vi "main(Test DQMH modules).vi"() -> ()   [LabVIEW 2018, in "Application.lvlib"] (continued)
      tunnel: [w268 w1259 w1272 w1282 w1301 w1434 w1477 w1534 w1590 w1602 w1614 w1623 w1648 w1678 w1708 w1775 w1790 w1813 w1836 w1860 w1894 w1913 w1932 w1951 w1983 w2014 w2039 w2068 w2104 w2124 w2147 w2181 w2198 w2224 w2256 w2294 w2331 w2381 w2418 w2465 w2520 w2593 w2663 w2734 w2805 w2876 w2947 w3018 w3090 w3163 w3239 w3318 w3398 w3479 w3561 w3607 w3648 w3689 w3730 w3771 w3812 w3853 w3894 w3935 w3976 w4017 w4058 w4099 w4140 w4181 w4222 w4263 w4304 w4345 w4386 w4427 w4468 w4509 w4550 w4591 w4632 w4673 w4714 w4755 w4796 w4837 w4878 w4919 w4960 w5001 w5042 w5083 w5124 w5165 w5206 w5247 w5288 w5329 w5370 w5411 w5452 w5493 w5534 w5575 w5616 w5657 w5698 w5739 w5780 w5821 w5862 w5903 w5944 w5985 w6026 w6064 1 ("DUT channel (1-11)") 1 ("DUT channel (1-11)") 1 ("DUT channel (1-11)") 1 ("DUT channel (1-11)") 1 ("DUT channel (1-11)") 1 ("DUT channel (1-11)") 2 ("DUT channel (1-11)") 2 ("DUT channel (1-11)") 2 ("DUT channel (1-11)") 2 ("DUT channel (1-11)") 2 ("DUT channel (1-11)") 2 ("DUT channel (1-11)") 3 ("DUT channel (1-11)") 3 ("DUT channel (1-11)") 3 ("DUT channel (1-11)") 3 ("DUT channel (1-11)") 3 ("DUT channel (1-11)") 3 ("DUT channel (1-11)") 4 ("DUT channel (1-11)") 4 ("DUT channel (1-11)") 4 ("DUT channel (1-11)") 4 ("DUT channel (1-11)") 4 ("DUT channel (1-11)") 4 ("DUT channel (1-11)") 5 ("DUT channel (1-11)") 5 ("DUT channel (1-11)") 5 ("DUT channel (1-11)") 5 ("DUT channel (1-11)") 5 ("DUT channel (1-11)") 5 ("DUT channel (1-11)") 6 ("DUT channel (1-11)") 6 ("DUT channel (1-11)") 6 ("DUT channel (1-11)") 6 ("DUT channel (1-11)") 6 ("DUT channel (1-11)") 6 ("DUT channel (1-11)") 7 ("DUT channel (1-11)") 7 ("DUT channel (1-11)") 7 ("DUT channel (1-11)") 7 ("DUT channel (1-11)") 7 ("DUT channel (1-11)") 7 ("DUT channel (1-11)") 8 ("DUT channel (1-11)") 8 ("DUT channel (1-11)") 8 ("DUT channel (1-11)") 8 ("DUT channel (1-11)") 8 ("DUT channel (1-11)") 8 ("DUT channel (1-11)") 9 ("DUT channel (1-11)") 9 ("DUT channel (1-11)") 9 ("DUT channel (1-11)") 9 ("DUT channel (1-11)") 9 ("DUT channel (1-11)") 9 ("DUT channel (1-11)") 10 ("DUT channel (1-11)") 10 ("DUT channel (1-11)") 10 ("DUT channel (1-11)") 10 ("DUT channel (1-11)") 10 ("DUT channel (1-11)") 10 ("DUT channel (1-11)")] -> w237
      tunnel: w236 -> [w269 w1259 w1272 w1282 w1301 w1434 w1477 w1534 w1590 w1602 w1614 w1623 w1648 w1678 w1708 w1775 w1790 w1813 w1836 w1860 w1894 w1913 w1932 w1951 w1983 w2014 w2039 w2068 w2104 w2124 w2147 w2181 w2198 w2224 w2256 w2294 w2331 w2381 w2418 w2465 _ _ _ _ _ _ _ _ _ _ _ _ _ _ _ w3607 w3648 w3689 w3730 w3771 w3812 w3853 w3894 w3935 w3976 w4017 w4058 w4099 w4140 w4181 w4222 w4263 w4304 w4345 w4386 w4427 w4468 w4509 w4550 w4591 w4632 w4673 w4714 w4755 w4796 w4837 w4878 w4919 w4960 w5001 w5042 w5083 w5124 w5165 w5206 w5247 w5288 w5329 w5370 w5411 w5452 w5493 w5534 w5575 w5616 w5657 w5698 w5739 w5780 w5821 w5862 w5903 w5944 w5985 w6026 w6064 _ _ _ _ _ _ _ _ _ _ _ _ _ _ _ _ _ _ _ _ _ _ _ _ _ _ _ _ _ _ _ _ _ _ _ _ _ _ _ _ _ _ _ _ _ _ _ _ _ _ _ _ _ _ _ _ _ _ _ _]
      tunnel: [w266 w1258 w1271 w1281 w1303 w1422 w1476 w1533 w1589 w1601 w1613 w1622 w1647 w1677 w1707 w1774 w1789 w1812 w1835 w1859 w1893 w1912 w1931 w1950 w1982 w2013 w2038 w2067 w2103 w2123 w2146 w2180 w2197 w2223 w2259 w2293 w2330 w2380 w2409 w2464 w2498 w2592 w2662 w2733 w2804 w2875 w2946 w3017 w3089 w3162 w3238 w3317 w3397 w3478 w3560 w3602 w3644 w3685 w3726 w3767 w3811 w3849 w3890 w3931 w3972 w4013 w4054 w4095 w4136 w4177 w4218 w4258 w4302 w4341 w4382 w4423 w4464 w4505 w4546 w4587 w4628 w4669 w4710 w4751 w4791 w4833 w4874 w4915 w4956 w4997 w5038 w5079 w5120 w5160 w5202 w5243 w5284 w5325 w5366 w5406 w5448 w5488 w5530 w5570 w5611 w5653 w5694 w5734 w5776 w5817 w5858 w5899 w5940 w5981 w6022 w6063 w6071 w6128 w6185 w6241 w6299 w6355 w6412 w6469 w6526 w6583 w6640 w6697 w6755 w6812 w6869 w6926 w6983 w7040 w7097 w7154 w7210 w7268 w7324 w7381 w7439 w7495 w7553 w7609 w7667 w7723 w7780 w7837 w7895 w7952 w8008 w8065 w8122 w8179 w8236 w8293 w8350 w8407 w8464 w8524 w8578 w8636 w8692 w8750 w8807 w8864 w8920 w8977 w9034 w9091 w9148 w9205 w9266 w9325 w9384 w9443] -> w235
      tunnel: w234 -> [w267 w1258 w1271 w1281 w1303 w1422 w1476 w1533 w1589 w1601 w1613 w1622 w1647 w1677 w1707 w1774 w1789 w1812 w1835 w1859 w1893 w1912 w1931 w1950 w1982 w2013 w2038 w2067 w2103 w2123 w2146 w2180 w2197 w2223 w2259 w2293 w2330 w2380 w2409 w2464 w2498 w2592 w2662 w2733 w2804 w2875 w2946 w3017 w3089 w3162 w3238 w3317 w3397 w3478 w3560 _ _ _ _ _ _ _ _ _ _ _ _ _ _ _ _ _ _ _ _ _ _ _ _ _ _ _ _ _ _ _ _ _ _ _ _ _ _ _ _ _ _ _ _ _ _ _ _ _ _ _ _ _ _ _ _ _ _ _ _ w6063 _ _ _ _ _ _ _ _ _ _ _ _ _ _ _ _ _ _ _ _ _ _ _ _ _ _ _ _ _ _ _ _ _ _ _ _ _ _ _ _ _ _ _ _ _ _ _ _ _ _ _ _ _ _ _ _ _ _ _ _]
      tunnel: w231 -> [w274 _ _ _ _ _ _ _ _ _ _ _ _ _ _ _ _ _ _ _ _ _ _ _ _ _ _ _ w2095 _ _ _ _ _ _ _ _ _ _ _ _ _ _ _ _ _ _ _ _ _ _ _ _ _ _ _ _ _ _ _ _ _ _ _ _ _ _ _ _ _ _ _ _ _ _ _ _ _ _ _ _ _ _ _ _ _ _ _ _ _ _ _ _ _ _ _ _ _ _ _ _ _ _ _ _ _ _ _ _ _ _ _ _ _ _ _ _ _ _ _ _ _ _ _ _ _ _ _ _ _ _ _ _ _ _ _ _ _ _ _ _ _ _ _ _ _ _ _ _ _ _ _ _ _ _ _ _ _ _ _ _ _ _ _ _ _ _ _ _ _ _ _ _ _ _ _]
      tunnel: [_ _ _ _ _ _ _ _ _ _ _ _ _ _ _ _ _ _ _ _ _ _ _ _ _ _ _ _ _ _ _ _ _ _ _ _ _ _ TRUE _ _ _ _ _ _ _ _ _ _ _ _ _ _ _ _ _ _ _ _ _ _ _ _ _ _ _ _ _ _ _ _ _ _ _ _ _ _ _ _ _ _ _ _ _ _ _ _ _ _ _ _ _ _ _ _ _ _ _ _ _ _ _ _ _ _ _ _ _ _ _ _ _ _ _ _ _ _ _ _ _ _ _ _ _ _ _ _ _ _ _ _ _ _ _ _ _ _ _ _ _ _ _ _ _ _ _ _ _ _ _ _ _ _ _ _ _ _ _ _ _ _ _ _ _ _ _ _ _ _ _ _ _ _ _ _ _] -> w230
      tunnel: [w270 w1257 w1265 w1277 w1299 w1432 "Test Completed!!!!" w1525 w1588 w1600 w1612 w1620 w1643 w1676 "Initialize Apps" w1752 w1785 w1808 w1831 w1854 w1888 w1907 w1926 w1945 w1971 w2008 w2035 w2064 w2090 "HV-60D ready!!!!!!!!!!!!!!!!" w2140 w2177 w2192 w2216 w2253 w2288 w2323 w2373 w2411 "Shorted Circuit Test" "Test Channel 1" "Test Channel 2" "Test Channel 3" "Test Channel 4" "Test Channel 5" "Test Channel 6" "Test Channel 7" "Test Channel 8" "Test Channel 9" "Test Channel 10" "Test Channel 10" "Test Channel 10" "Test Channel 10" "Test Channel 10" "Test Channel 10" w3605 w3647 w3688 w3729 w3770 w3809 w3852 w3893 w3934 w3975 w4016 w4057 w4098 w4139 w4180 w4221 w4262 w4301 w4344 w4385 w4426 w4467 w4508 w4549 w4590 w4631 w4672 w4713 w4754 w4795 w4836 w4877 w4918 w4959 w5000 w5041 w5082 w5123 w5164 w5205 w5246 w5287 w5328 w5369 w5410 w5451 w5492 w5533 w5574 w5615 w5656 w5697 w5738 w5779 w5820 w5861 w5902 w5943 w5984 w6025 w6062 w6080 w6137 w6194 w6251 w6308 w6365 w6422 w6479 w6536 w6593 w6650 w6707 w6764 w6821 w6879 w6936 w6993 w7050 w7107 w7164 w7221 w7278 w7335 w7392 w7449 w7506 w7563 w7620 w7677 w7734 w7791 w7848 w7905 w7962 w8019 w8076 w8133 w8191 w8247 w8304 w8361 w8418 w8475 w8532 w8589 w8646 w8705 w8760 w8817 w8874 w8931 w8988 w9046 w9102 w9159 w9216 w9276 w9335 w9394 w9453] -> w227
      tunnel: w226 -> [w271 w1257 w1265 w1277 w1299 w1432 _ _ w1588 w1600 w1612 w1620 w1643 w1676 _ w1752 w1785 w1808 w1831 w1854 w1888 w1907 w1926 w1945 w1971 w2008 w2035 w2064 w2090 _ w2140 w2177 w2192 w2216 w2253 w2288 w2323 w2373 w2411 _ _ _ _ _ _ _ _ _ _ _ _ _ _ _ _ w3604 w3646 w3687 w3728 w3769 w3808 w3851 w3892 w3933 w3974 w4015 w4056 w4097 w4138 w4179 w4220 w4261 w4300 w4343 w4384 w4425 w4466 w4507 w4548 w4589 w4630 w4671 w4712 w4753 w4794 w4835 w4876 w4917 w4958 w4999 w5040 w5081 w5122 w5163 w5204 w5245 w5286 w5327 w5368 w5409 w5450 w5491 w5532 w5573 w5614 w5655 w5696 w5737 w5778 w5819 w5860 w5901 w5942 w5983 w6024 w6062 _ _ _ _ _ _ _ _ _ _ _ _ _ _ _ _ _ _ _ _ _ _ _ _ _ _ _ _ _ _ _ _ _ _ _ _ _ _ _ _ _ _ _ _ _ _ _ _ _ _ _ _ _ _ _ _ _ _ _ _]
      tunnel: w224 -> [_ _ _ _ _ _ w1456 _ _ _ _ _ _ _ _ _ _ _ _ _ _ _ _ _ _ _ _ _ _ _ _ _ _ _ _ _ _ _ _ _ _ _ _ _ _ _ _ _ _ _ _ _ _ _ _ _ _ _ _ _ _ _ _ _ _ _ _ _ _ _ _ _ _ _ _ _ _ _ _ _ _ _ _ _ _ _ _ _ _ _ _ _ _ _ _ _ _ _ _ _ _ _ _ _ _ _ _ _ _ _ _ _ _ _ _ _ _ _ _ _ _ _ _ _ _ _ _ _ _ _ _ _ _ _ _ _ _ _ _ _ _ _ _ _ _ _ _ _ _ _ _ _ _ _ _ _ _ _ _ _ _ _ _ _ _ _ _ _ _ _ _ _ _ _ _ _]
      frame "Apps.WaitForEvent", Default {
        n141 = event shown="[7] \"Settings\": Value Change" {
          selector: w283 -> [_ w311 _ _ _ _ _ _ _ _ _ _ _ _ _ _ _ _ _ _ _ _ _ _ _ _ _ _ _ _ _ _ _ _ _ _ _ _ _ _ _ _]
          dyn-events: [_ w311 _ _ _ _ _ _ _ _ _ _ _ _ _ _ _ _ _ _ _ _ _ _ _ _ _ _ _ _ _ _ _ _ _ _ _ _ _ _ _ _] -> w282
          timeout: w272 -> [_ _ _ _ _ _ _ _ _ _ _ _ _ _ _ _ _ _ _ _ _ _ _ _ _ _ _ _ _ _ _ _ _ _ _ _ _ _ _ _ _ _]
          tunnel: [w290 w306 w324 w347 w362 w380 w397 w422 w433 w451 w459 w481 w500 w517 w529 w550 w572 w607 w626 w643 w667 w686 w705 w734 w774 w794 w822 w930 w961 w984 w1005 w1026 w1047 w1068 w1089 w1110 w1131 w1152 w1173 w1189 w1214 w1239] -> w284
          tunnel: w272 -> [w290 w306 w325 w347 w362 w380 w396 w422 w433 w451 w459 w481 w500 w517 w529 w550 w572 w607 w626 w643 w667 w686 w705 w734 w774 w794 w822 w930 w961 w984 w1005 w1026 w1047 w1068 w1089 w1110 w1131 w1152 w1173 w1189 w1214 w1239]
          tunnel: [w294 w310 _ w338 _ w377 w386 w416 w427 w446 w457 w476 w495 w509 w525 w548 w570 w600 w621 w640 w665 w684 w703 w728 w766 w788 w818 w929 w958 w982 w1003 w1024 w1045 w1066 w1087 w1108 w1129 w1150 w1171 w1187 w1211 w1236] -> w280
          tunnel: w279 -> [w288 w310 _ w340 _ w379 w401 w417 w429 w450 w456 w475 w494 w510 w524 w547 w569 w599 w620 w639 w664 w683 w702 w727 w768 w792 w817 w928 w959 w983 w1004 w1025 w1046 w1067 w1088 w1109 w1130 w1151 w1172 w1186 w1210 w1237]
          tunnel: w278 -> [w291 w304 w326 w342 _ w368 w403 w420 w430 w449 w462 w480 w499 _ w519 w555 w576 w604 w625 w651 w670 w689 w710 w731 w773 w795 w819 w918 w955 w979 w1000 w1021 w1042 w1063 w1084 w1106 w1126 w1147 w1168 w1180 w1205 w1230]
          tunnel: [w295 w313 w331 w346 w361 w376 w402 w421 w431 w444 w458 w478 w496 w516 w526 w549 w571 w601 w622 w642 w666 w685 w704 w733 w769 w789 w820 w931 w954 w977 w998 w1019 w1040 w1061 w1082 w1104 w1124 w1145 w1166 w1188 w1213 w1238] -> w277
          tunnel: w276 -> [w295 w313 w331 w346 w361 w376 w402 w421 w431 w444 w458 w478 w496 w516 w526 w549 w571 w601 w622 w642 w666 w685 w704 w733 w769 _ w821 w931 w954 w977 w998 w1019 w1040 w1061 w1082 w1104 w1124 w1145 w1166 w1188 w1213 w1238]
          tunnel: w275 -> [_ _ _ w336 _ _ w389 _ _ _ _ _ _ _ _ _ _ _ _ _ _ _ _ _ _ _ _ _ _ w976 w995 w1015 w1036 w1057 w1078 w1099 w1120 w1141 w1162 _ _ _]
          tunnel: w273 -> [w293 w312 _ _ _ _ _ _ _ _ w455 w474 w493 _ w523 w546 w568 w598 w619 w638 w663 w682 w701 w726 w765 w790 w815 w927 _ _ _ _ _ _ _ _ _ _ _ w1185 w1212 w1235]
          tunnel: w274 -> [_ _ _ _ _ _ _ _ _ _ _ _ _ _ _ _ _ _ _ _ _ _ _ _ _ _ _ _ _ _ _ _ _ _ _ _ _ _ _ _ _ _]
          tunnel: w269 -> [w286 w308 w329 w344 w359 w374 w391 w414 w425 w442 w453 w472 w491 w514 w521 w544 _ w596 w617 w636 w661 w680 w699 w723 w763 w784 w812 w914 w952 _ _ _ _ _ _ _ _ _ _ w1183 w1208 w1233]
          tunnel: w271 -> [w287 _ w330 w345 w360 w375 _ _ w426 w443 w454 w473 w492 w515 w522 w545 w567 w597 w618 w637 w662 w681 w700 w725 w764 w785 w813 w915 w953 w972 w993 w1014 w1035 w1056 w1077 w1098 w1119 w1140 w1161 w1184 w1209 w1234]
          tunnel: [w287 "Wait for JIG lock" w330 w345 w360 w375 "Start Auto Test" "Settings" w426 w443 w454 w473 w492 w515 w522 w545 w567 w597 w618 w637 w662 w681 w700 w725 w764 w785 w813 w915 w953 w972 w993 w1014 w1035 w1056 w1077 w1098 w1119 w1140 w1161 w1184 w1209 w1234] -> w270
          tunnel: [w286 w308 w329 w344 w359 w374 w391 w414 w425 w442 w453 w472 w491 w514 w521 w544 w564 w596 w617 w636 w661 w680 w699 w723 w763 w784 w811 w914 w952 1 ("DUT channel (1-11)") 2 ("DUT channel (1-11)") 3 ("DUT channel (1-11)") 4 ("DUT channel (1-11)") 5 ("DUT channel (1-11)") 6 ("DUT channel (1-11)") 7 ("DUT channel (1-11)") 8 ("DUT channel (1-11)") 9 ("DUT channel (1-11)") 10 ("DUT channel (1-11)") w1183 w1208 w1233] -> w268
          tunnel: w267 -> [w285 w307 w328 w343 w358 w373 w390 w413 w424 w441 w452 w471 w490 w513 w520 w543 w566 w595 w616 w635 w660 w679 w698 _ w762 w783 w807 w913 w951 w970 w991 w1012 w1033 w1054 w1075 w1096 w1117 w1138 w1159 w1179 w1204 w1229]
          tunnel: [w285 w307 w328 w343 w358 w373 w390 w413 w424 w441 w452 w471 w490 w513 w520 w543 w566 w595 w616 w635 w660 w679 w698 w719 w762 w783 w806 w913 w951 w970 w991 w1012 w1033 w1054 w1075 w1096 w1117 w1138 w1159 w1179 w1204 w1229] -> w266
          tunnel: w265 -> [_ _ _ _ _ _ _ _ _ _ _ _ _ _ _ _ _ _ _ _ _ _ _ _ _ _ w810 _ _ _ _ _ _ _ _ _ _ _ _ _ _ _]
          event Timeout {
            n142 = event-data() -> ()  [unwired: 1 in, 1 out]
            n143 = disable-structure shown="LOGGING==TRUE" {
              disable-tunnel: w293 -> [w296 _]
              frame condition #0 (active) {
                n144 = Empty String/Path?(string/path=w296) -> (empty?=w303:bool)
                n145 = Select(t="Quece timeout", s=w303, f=w296) -> (s? t:f=w301:string)
                n146 = Format Into String(format string=": %s", initial string=w301, "UI timeout") -> (resulting string=w298:string)  [unwired: 1 in, 1 out]
                n147 = call "string log (SubVI).vi"("Enum"=enum16{"Init", "Log", "Read"}."Log", "state Name"=w298) -> ()  [unwired: 8 in, 2 out]
              }
              frame condition #1 {
              }
            }
            n148 = call "App enquece.vi"("command"="Apps.WaitingForTrigger", "queue in"=w291) -> ("error out"=w289:errorcluster)  [unwired: 8 in, 1 out]
            n149 = Merge Errors(w288, w289) -> (w294:errorcluster)
          }
          event "Test": Value Change {
            n150 = event-data() -> ()  [unwired: 1 in, 2 out]
            n151 = disable-structure shown="Default" {
              disable-tunnel: w312 -> [w316 _]
              frame condition #0 (active) {
                n152 = Empty String/Path?(string/path=w316) -> (empty?=w323:bool)
                n153 = Select(t="Quece timeout", s=w323, f=w316) -> (s? t:f=w321:string)
                n154 = Format Into String(format string=": %s", initial string=w321, "Test") -> (resulting string=w318:string)  [unwired: 1 in, 1 out]
                n155 = call "string log (SubVI).vi"("Enum"=enum16{"Init", "Log", "Read"}."Log", "state Name"=w318) -> ()  [unwired: 8 in, 2 out]
              }
              frame condition #1 {
              }
            }
            n156 = call "App enquece.vi"("command"="Apps.AutoMode", "queue in"=w304) -> ()  [unwired: 8 in, 2 out]
            n157 = disable-structure shown="Disabled" {
              frame Disabled {
                n158 = Select(t=100, f=-1) -> ()  [unwired: 1 in, 1 out]
              }
              frame Enabled {
              }
            }
          }
          event "Auto/Man": Value Change {
            n159 = event-data() -> ("NewVal"=w327:bool)  [unwired: 1 in, 5 out]
            n160 = case shown="True" w327 {
              tunnel: w326 -> [_ w334]
              tunnel: [-1 w333] -> w324
              tunnel: w325 -> [_ w333]
              frame False {
              }
              frame True {
                n161 = call "App enquece.vi"("command"="Apps.AutoMode", "queue in"=w334) -> ()  [unwired: 8 in, 2 out]
              }
            }
          }
          event "Test Single DRV": Value Change {
            n162 = event-data() -> ()  [unwired: 1 in, 1 out]
            n163 = case shown="1.." "DRV number" {
              selector: "DRV number" -> [_ w350]
              tunnel: ["MEAS.AllRelaysOFF" w353] -> w341
              tunnel: w336 -> [w348 _]
              frame 0, Default {
                n164 = call "reset DRV UI (SubVI).vi"("Ref  in"=w348) -> ()  [unwired: 9 in, 2 out]
              }
              frame 1.. {
                n165 = Format Into String(format string="%d%s", initial string="Test DRV ", w350, "A" ("input 3")) -> (resulting string=w353:string)  [unwired: 1 in, 1 out]
              }
            }
            n166 = call "App enquece.vi"("command"=w341, "queue in"=w342) -> ("error out"=w339:errorcluster)  [unwired: 8 in, 1 out]
            n167 = Merge Errors(w340, w339) -> (w338:errorcluster)
          }
          event "DMM query": Value Change {
            n168 = event-data() -> ()  [unwired: 1 in, 6 out]
            n169 = flat-sequence {
              tunnel: [w365] -> w356
              frame #0 {
                w363 = ""
                n170 = Wait (ms)(milliseconds to wait=u32 100) -> ()  [unwired: 1 out]
                n171 = local write "DMM func?"(w363) -> ()
                n172 = local write "DMM range?"(w363) -> ()
                n173 = xnode "Error Ring"() -> ("error out"=w365:errorcluster)
              }
            }
            n174 = call "Query func.vi"("error in"=w356) -> ("String"=→"DMM func?":string)  [unwired: 8 in, 2 out]
            n175 = call "query range.vi"("error in"=w356) -> ("String"=→"DMM range?":string)  [unwired: 8 in, 2 out]
          }
          event "VIEW": Value Change {
            n176 = event-data() -> ()  [unwired: 1 in, 1 out]
            n177 = disable-structure shown="Disabled" {
              frame Disabled {
                n178 = Initialize Array(FALSE, 6 ("dimension size"), 10 ("dimension size")) -> (w381:bool[][])
                n179 = local write "Short DRV"(w381) -> ()
              }
              frame Enabled {
              }
            }
            n180 = call "App enquece.vi"("command"="Apps.UI Update 1", "queue in"=w368) -> ()  [unwired: 8 in, 2 out]
            n181 = invoke class="VI" method="FP.Open"("State"=T18."Hidden") -> (error out=w372:errorcluster)  [unwired: 4 in, 4 out]
            n182 = call "View DRV data.vi"("error in (no error)"=w372) -> ("error out"=w371:errorcluster)  [unwired: 10 in]
            n183 = invoke class="VI" method="FP.Open"(error in=w371, "State"=T18."Standard") -> (error out=w378:errorcluster)  [unwired: 3 in, 4 out]
            n184 = Merge Errors(w379, w378) -> (w377:errorcluster)
          }
          event User Event {
            # "#HungNotes:\nStart HV60D from this frame (check new board  installed)"
            # "Stop Timeout event"
            n185 = event-data() -> ("new board?"=w395:bool, "new trigger"=→"new Trigger?":bool, "last trigger"=→"last Trigger?":bool)  [unwired: 1 in, 1 out]
            "New board?" <- w395
            n186 = call "reset DRV UI (SubVI).vi"("Ref  in"=w389) -> ()  [unwired: 9 in, 2 out]
            n187 = case shown="True" w395 {
              tunnel: w403 -> [_ w409]
              tunnel: [_ w408] -> w388
              frame False {
              }
              frame True {
                n188 = call "FGV DUT steps.vi"("Enum"=enum16{"write", "read"}."read") -> ("Steps OUT"=w406:string[])  [unwired: 10 in]
                n189 = Array Subset(array=w406, index=2) -> (w404:string[])  [unwired: 1 in]
                n190 = for {
                  tunnel: [w412] -> w408 mode=indexing
                  tunnel: w409 -> [w411]
                  tunnel: w404 -> [w410] mode=indexing
                  n191 = call "App enquece.vi"("command"=w410, "queue in"=w411) -> ("error out"=w412:errorcluster)  [unwired: 8 in, 1 out]
                }
              }
            }
            n192 = Merge Errors(w401, w388) -> (w387:errorcluster)
            n193 = Select(t=-1, s=w395, f=w396) -> (s? t:f=w397:i32)
            n194 = local write "Report file Name"("") -> ()
            n195 = control-ref of="DRV 61"() -> (w393:refnum<vi>)
            n196 = property class="ColBox"(reference=w393, error in=w387, "Value"=u32 10000536 ("DRV 1")) -> (error out=w386:errorcluster)  [unwired: 1 out]
          }
          event "Settings": Value Change {
            n197 = event-data() -> ()  [unwired: 1 in, 6 out]
            n198 = call "App enquece.vi"("command"="INIT.Read DRV code", "queue in"=w420) -> ("error out"=w418:errorcluster)  [unwired: 8 in, 1 out]
            n199 = Merge Errors(w417, w418) -> (w416:errorcluster)
          }
          event Panel Close? {
            n200 = event-data() -> ()  [unwired: 1 in, 4 out]
            n201 = disable-structure shown="Disabled" {
              disable-tunnel: [w434 TRUE] -> w423
              frame Disabled {
                n202 = Two Button Dialog(message="Do you want to exit progam") -> (T button?=w434:bool)  [unwired: 2 in]
              }
              frame Enabled {
              }
            }
            n203 = case shown="True" w423 {
              tunnel: w430 -> [_ w439]
              tunnel: [_ w437] -> w428
              frame False {
              }
              frame True {
                n204 = call "App enquece.vi"("Priority Enquece"=TRUE, "command"="Apps.Exit", "queue in"=w439) -> ("error out"=w437:errorcluster)  [unwired: 7 in, 1 out]
              }
            }
            n205 = Merge Errors(w429, w428) -> (w427:errorcluster)
            n206 = event-data("Discard?"=TRUE) -> ()  [unwired: 1 in, 1 out]
          }
          event "Exit": Value Change {
            n207 = event-data() -> ()  [unwired: 1 in, 1 out]
            n208 = call "App enquece.vi"("Priority Enquece"=TRUE, "command"="Apps.Exit", "queue in"=w449) -> ("error out"=w448:errorcluster)  [unwired: 7 in, 1 out]
            n209 = Merge Errors(w450, w448) -> (w446:errorcluster)
          }
          event "check connected": Value Change {
            n210 = event-data() -> ()  [unwired: 1 in, 1 out]
            n211 = disable-structure shown="LOGGING==TRUE" {
              disable-tunnel: w455 -> [w463 _]
              frame condition #0 (active) {
                n212 = Empty String/Path?(string/path=w463) -> (empty?=w470:bool)
                n213 = Select(t="Quece timeout", s=w470, f=w463) -> (s? t:f=w468:string)
                n214 = Format Into String(format string=": %s", initial string=w468, "Check connected") -> (resulting string=w465:string)  [unwired: 1 in, 1 out]
                n215 = call "string log (SubVI).vi"("Enum"=enum16{"Init", "Log", "Read"}."Log", "state Name"=w465) -> ()  [unwired: 8 in, 2 out]
              }
              frame condition #1 {
              }
            }
            n216 = call "App enquece.vi"("command"="MEAS.Read EMIC connected", "queue in"=w462) -> ("error out"=w460:errorcluster)  [unwired: 8 in, 1 out]
            n217 = Merge Errors(w456, w460) -> (w457:errorcluster)
          }
          event "Open COM eMIC": Value Change {
            n218 = event-data() -> ()  [unwired: 1 in, 1 out]
            n219 = disable-structure shown="LOGGING==TRUE" {
              disable-tunnel: w474 -> [w482 _]
              frame condition #0 (active) {
                n220 = Empty String/Path?(string/path=w482) -> (empty?=w489:bool)
                n221 = Select(t="Quece timeout", s=w489, f=w482) -> (s? t:f=w487:string)
                n222 = Format Into String(format string=": %s", initial string=w487, "Open COM eMIC") -> (resulting string=w484:string)  [unwired: 1 in, 1 out]
                n223 = call "string log (SubVI).vi"("Enum"=enum16{"Init", "Log", "Read"}."Log", "state Name"=w484) -> ()  [unwired: 8 in, 2 out]
              }
              frame condition #1 {
              }
            }
            n224 = call "App enquece.vi"("command"="INIT.Open COM EMIC", "queue in"=w480) -> ("error out"=w479:errorcluster)  [unwired: 8 in, 1 out]
            n225 = Merge Errors(w475, w479) -> (w476:errorcluster)
          }
          event "Read trigger": Value Change {
            n226 = event-data() -> ()  [unwired: 1 in, 1 out]
            n227 = disable-structure shown="LOGGING==TRUE" {
              disable-tunnel: w493 -> [w501 _]
              frame condition #0 (active) {
                n228 = Empty String/Path?(string/path=w501) -> (empty?=w508:bool)
                n229 = Select(t="Quece timeout", s=w508, f=w501) -> (s? t:f=w506:string)
                n230 = Format Into String(format string=": %s", initial string=w506, "Read Trigger") -> (resulting string=w503:string)  [unwired: 1 in, 1 out]
                n231 = call "string log (SubVI).vi"("Enum"=enum16{"Init", "Log", "Read"}."Log", "state Name"=w503) -> ()  [unwired: 8 in, 2 out]
              }
              frame condition #1 {
              }
            }
            n232 = call "App enquece.vi"("command"="MEAS.Read TRIGGER", "queue in"=w499) -> ("error out"=w497:errorcluster)  [unwired: 8 in, 1 out]
            n233 = Merge Errors(w494, w497) -> (w495:errorcluster)
          }
          event "Set trigger value": Value Change {
            n234 = event-data() -> ()  [unwired: 1 in, 6 out]
            n235 = call "SET trigger value.vi"("Boolean"="set value") -> ("error out"=w511:errorcluster)  [unwired: 10 in]
            n236 = Merge Errors(w510, w511) -> (w509:errorcluster)
          }
          event "Read Optos": Value Change {
            n237 = event-data() -> ()  [unwired: 1 in, 1 out]
            n238 = disable-structure shown="LOGGING==TRUE" {
              disable-tunnel: w523 -> [w535 _]
              frame condition #0 (active) {
                n239 = Empty String/Path?(string/path=w535) -> (empty?=w542:bool)
                n240 = Select(t="Quece timeout", s=w542, f=w535) -> (s? t:f=w540:string)
                n241 = Format Into String(format string=": %s", initial string=w540, "Read Optos") -> (resulting string=w537:string)  [unwired: 1 in, 1 out]
                n242 = call "string log (SubVI).vi"("Enum"=enum16{"Init", "Log", "Read"}."Log", "state Name"=w537) -> ()  [unwired: 8 in, 2 out]
              }
              frame condition #1 {
              }
            }
            n243 = flat-sequence {
              tunnel: w519 -> [w530]
              tunnel: [w530] -> w518
              frame #0 {
                n244 = Initialize Array(FALSE, 6 ("dimension size"), 10 ("dimension size")) -> (w534:bool[][])
                n245 = local write "Short DRV"(w534) -> ()
              }
            }
            n246 = call "App enquece.vi"("command"="MEAS.Read Optos", "queue in"=w518) -> ("error out"=w527:errorcluster)  [unwired: 8 in, 1 out]
            n247 = Merge Errors(w524, w527) -> (w525:errorcluster)
          }
          event "Select DMM's Current Input": Value Change {
            n248 = event-data() -> ()  [unwired: 1 in, 1 out]
            n249 = disable-structure shown="LOGGING==TRUE" {
              disable-tunnel: w546 -> [w556 _]
              frame condition #0 (active) {
                n250 = Empty String/Path?(string/path=w556) -> (empty?=w563:bool)
                n251 = Select(t="Quece timeout", s=w563, f=w556) -> (s? t:f=w561:string)
                n252 = Format Into String(format string=": %s", initial string=w561, "DMM Current Input") -> (resulting string=w558:string)  [unwired: 1 in, 1 out]
                n253 = call "string log (SubVI).vi"("Enum"=enum16{"Init", "Log", "Read"}."Log", "state Name"=w558) -> ()  [unwired: 8 in, 2 out]
              }
              frame condition #1 {
              }
            }
            n254 = To Variant(anything="mux2-1(DMM I) encode") -> (Variant=w552:variant)
            n255 = call "App enquece.vi"("command data"=w552, "command"="MEAS.Sel Input Current", "queue in"=w555) -> ("error out"=w551:errorcluster)  [unwired: 7 in, 1 out]
            n256 = Merge Errors(w547, w551) -> (w548:errorcluster)
          }
          event "DEMUX 1-10": Value Change {
            n257 = event-data() -> ()  [unwired: 1 in, 1 out]
            n258 = disable-structure shown="LOGGING==TRUE" {
              disable-tunnel: w568 -> [w587 _]
              frame condition #0 (active) {
                n259 = Empty String/Path?(string/path=w587) -> (empty?=w594:bool)
                n260 = Select(t="Quece timeout", s=w594, f=w587) -> (s? t:f=w592:string)
                n261 = Format Into String(format string=": %s", initial string=w592, "demux1-10") -> (resulting string=w589:string)  [unwired: 1 in, 1 out]
                n262 = call "string log (SubVI).vi"("Enum"=enum16{"Init", "Log", "Read"}."Log", "state Name"=w589) -> ()  [unwired: 8 in, 2 out]
              }
              frame condition #1 {
              }
            }
            n263 = To Variant(anything="demux1_10(x6)_encode") -> (Variant=w574:variant)
            n264 = case shown="\"demux1_10_channel0\", Default" "demux1_10(x6)_encode" {
              tunnel: [_ 1 ("DUT channel (1-11)") 2 ("DUT channel (1-11)") 3 ("DUT channel (1-11)") 4 ("DUT channel (1-11)") 5 ("DUT channel (1-11)") 6 ("DUT channel (1-11)") 7 ("DUT channel (1-11)") 8 ("DUT channel (1-11)") 9 ("DUT channel (1-11)") 10 ("DUT channel (1-11)")] -> w564
              frame "demux1_10_channel0", Default {
              }
              frame "demux1_10_channel1" {
              }
              frame "demux1_10_channel2" {
              }
              frame "demux1_10_channel3" {
              }
              frame "demux1_10_channel4" {
              }
              frame "demux1_10_channel5" {
              }
              frame "demux1_10_channel6" {
              }
              frame "demux1_10_channel7" {
              }
              frame "demux1_10_channel8" {
              }
              frame "demux1_10_channel9" {
              }
              frame "demux1_10_channel10" {
              }
            }
            n265 = call "App enquece.vi"("command data"=w574, "command"="MEAS.demux1-10", "queue in"=w576) -> ("error out"=w573:errorcluster)  [unwired: 7 in, 1 out]
            n266 = Merge Errors(w569, w573) -> (w570:errorcluster)
          }
          event "eMIC": Value Change {
            n267 = event-data() -> ()  [unwired: 1 in, 1 out]
            n268 = disable-structure shown="LOGGING==TRUE" {
              disable-tunnel: w598 -> [w608 _]
              frame condition #0 (active) {
                n269 = Empty String/Path?(string/path=w608) -> (empty?=w615:bool)
                n270 = Select(t="Quece timeout", s=w615, f=w608) -> (s? t:f=w613:string)
                n271 = Format Into String(format string=": %s", initial string=w613, "eMIC") -> (resulting string=w610:string)  [unwired: 1 in, 1 out]
                n272 = call "string log (SubVI).vi"("Enum"=enum16{"Init", "Log", "Read"}."Log", "state Name"=w610) -> ()  [unwired: 8 in, 2 out]
              }
              frame condition #1 {
              }
            }
            n273 = To Variant(anything="eMIC 6 values") -> (Variant=w602:variant)
            n274 = call "App enquece.vi"("command data"=w602, "command"="MEAS.eMIC", "queue in"=w604) -> ("error out"=w606:errorcluster)  [unwired: 7 in, 1 out]
            n275 = Merge Errors(w599, w606) -> (w600:errorcluster)
          }
          event "connect DMM": Value Change {
            n276 = event-data() -> ()  [unwired: 1 in, 1 out]
            n277 = disable-structure shown="LOGGING==TRUE" {
              disable-tunnel: w619 -> [w627 _]
              frame condition #0 (active) {
                n278 = Empty String/Path?(string/path=w627) -> (empty?=w634:bool)
                n279 = Select(t="Quece timeout", s=w634, f=w627) -> (s? t:f=w632:string)
                n280 = Format Into String(format string=": %s", initial string=w632, "Connect DMM") -> (resulting string=w629:string)  [unwired: 1 in, 1 out]
                n281 = call "string log (SubVI).vi"("Enum"=enum16{"Init", "Log", "Read"}."Log", "state Name"=w629) -> ()  [unwired: 8 in, 2 out]
              }
              frame condition #1 {
              }
            }
            n282 = call "App enquece.vi"("command"="INIT.Open COM DMM", "queue in"=w625) -> ("error out"=w624:errorcluster)  [unwired: 8 in, 1 out]
            n283 = Merge Errors(w620, w624) -> (w621:errorcluster)
          }
          event "config DMM": Value Change {
            n284 = event-data() -> ()  [unwired: 1 in, 1 out]
            n285 = disable-structure shown="LOGGING==TRUE" {
              disable-tunnel: w638 -> [w652 _]
              frame condition #0 (active) {
                n286 = Empty String/Path?(string/path=w652) -> (empty?=w659:bool)
                n287 = Select(t="Quece timeout", s=w659, f=w652) -> (s? t:f=w657:string)
                n288 = Format Into String(format string=": %s", initial string=w657, "config DMM") -> (resulting string=w654:string)  [unwired: 1 in, 1 out]
                n289 = call "string log (SubVI).vi"("Enum"=enum16{"Init", "Log", "Read"}."Log", "state Name"=w654) -> ()  [unwired: 8 in, 2 out]
              }
              frame condition #1 {
              }
            }
            n290 = Bundle By Name(cluster=T19 {"DMM config cluster"={"DCV range"=0.0, "DCI range"=0.0, "Detector Rate"=0}, "mux2-1(DMM I) encode"=enum."DMM I (0.5)"} ("DMM all config"), "DMM config cluster.DCV range"="DCV range", "DMM config cluster.DCI range"="DCI range", "DMM config cluster.Detector Rate"="Detector Rate") -> (w646:T19)
            n291 = To Variant(anything=w646) -> (Variant=w644:variant)
            n292 = call "App enquece.vi"("command data"=w644, "command"="MEAS.Set DMM config", "queue in"=w651) -> ("error out"=w641:errorcluster)  [unwired: 7 in, 1 out]
            n293 = Merge Errors(w639, w641) -> (w640:errorcluster)
          }
          event "DMM read dual value": Value Change {
            n294 = event-data() -> ()  [unwired: 1 in, 1 out]
            n295 = disable-structure shown="LOGGING==TRUE" {
              disable-tunnel: w663 -> [w671 _]
              frame condition #0 (active) {
                n296 = Empty String/Path?(string/path=w671) -> (empty?=w678:bool)
                n297 = Select(t="Quece timeout", s=w678, f=w671) -> (s? t:f=w676:string)
                n298 = Format Into String(format string=": %s", initial string=w676, "DMM read dual value") -> (resulting string=w673:string)  [unwired: 1 in, 1 out]
                n299 = call "string log (SubVI).vi"("Enum"=enum16{"Init", "Log", "Read"}."Log", "state Name"=w673) -> ()  [unwired: 8 in, 2 out]
              }
              frame condition #1 {
              }
            }
            n300 = call "App enquece.vi"("command"="MEAS.DMM dual read", "queue in"=w670) -> ("error out"=w668:errorcluster)  [unwired: 8 in, 1 out]
            n301 = Merge Errors(w664, w668) -> (w665:errorcluster)
          }
          event "Reset JIG": Value Change {
            n302 = event-data() -> ()  [unwired: 1 in, 1 out]
            n303 = disable-structure shown="LOGGING==TRUE" {
              disable-tunnel: w682 -> [w690 _]
              frame condition #0 (active) {
                n304 = Empty String/Path?(string/path=w690) -> (empty?=w697:bool)
                n305 = Select(t="Quece timeout", s=w697, f=w690) -> (s? t:f=w695:string)
                n306 = Format Into String(format string=": %s", initial string=w695, "reset JIG") -> (resulting string=w692:string)  [unwired: 1 in, 1 out]
                n307 = call "string log (SubVI).vi"("Enum"=enum16{"Init", "Log", "Read"}."Log", "state Name"=w692) -> ()  [unwired: 8 in, 2 out]
              }
              frame condition #1 {
              }
            }
            n308 = call "App enquece.vi"("command"="MEAS.Reset JIG", "queue in"=w689) -> ("error out"=w687:errorcluster)  [unwired: 8 in, 1 out]
            n309 = Merge Errors(w683, w687) -> (w684:errorcluster)
          }
          event "TurnON/OFF +5V": Value Change {
            n310 = event-data() -> ()  [unwired: 1 in, 1 out]
            n311 = disable-structure shown="LOGGING==TRUE" {
              disable-tunnel: w701 -> [w711 _]
              frame condition #0 (active) {
                n312 = Empty String/Path?(string/path=w711) -> (empty?=w718:bool)
                n313 = Select(t="Quece timeout", s=w718, f=w711) -> (s? t:f=w716:string)
                n314 = Format Into String(format string=": %s", initial string=w716, "ON/OFF +5V") -> (resulting string=w713:string)  [unwired: 1 in, 1 out]
                n315 = call "string log (SubVI).vi"("Enum"=enum16{"Init", "Log", "Read"}."Log", "state Name"=w713) -> ()  [unwired: 8 in, 2 out]
              }
              frame condition #1 {
              }
            }
            n316 = To Variant(anything="5V Value") -> (Variant=w707:variant)
            n317 = call "App enquece.vi"("command data"=w707, "command"="MEAS.Turn+5V", "queue in"=w710) -> ("error out"=w709:errorcluster)  [unwired: 7 in, 1 out]
            n318 = Merge Errors(w702, w709) -> (w703:errorcluster)
          }
          event "mux 6-1": Value Change {
            n319 = event-data() -> ()  [unwired: 1 in, 1 out]
            n320 = disable-structure shown="LOGGING==TRUE" {
              disable-tunnel: w726 -> [w754 _]
              frame condition #0 (active) {
                n321 = Empty String/Path?(string/path=w754) -> (empty?=w761:bool)
                n322 = Select(t="Quece timeout", s=w761, f=w754) -> (s? t:f=w759:string)
                n323 = Format Into String(format string=": %s", initial string=w759, "mux6-1") -> (resulting string=w756:string)  [unwired: 1 in, 1 out]
                n324 = call "string log (SubVI).vi"("Enum"=enum16{"Init", "Log", "Read"}."Log", "state Name"=w756) -> ()  [unwired: 8 in, 2 out]
              }
              frame condition #1 {
              }
            }
            n325 = Decrement(x=w723) -> (x-1=w722:i32)
            n326 = Multiply(x=w722, y=6) -> (x*y=w720:i32)
            n327 = case shown="\"mux6_1_channel6_3\"" "mux 6-1 data" {
              tunnel: w720 -> [_ w738 w741 w744 w747 w750 w753]
              tunnel: [0 w736 w739 w742 w745 w748 w751] -> w719
              frame "mux6-1_channel0", Default {
              }
              frame "mux6_1_channel1_3" {
                n328 = Add(x=w738, y=0) -> (x+y=w736:i32)
              }
              frame "mux6_1_channel2_3" {
                n329 = Add(x=w741, y=1) -> (x+y=w739:i32)
              }
              frame "mux6_1_channel3_3" {
                n330 = Add(x=w744, y=2) -> (x+y=w742:i32)
              }
              frame "mux6_1_channel4_3" {
                n331 = Add(x=w747, y=3) -> (x+y=w745:i32)
              }
              frame "mux6_1_channel5_3" {
                n332 = Add(x=w750, y=4) -> (x+y=w748:i32)
              }
              frame "mux6_1_channel6_3" {
                n333 = Add(x=w753, y=5) -> (x+y=w751:i32)
              }
            }
            n334 = To Variant(anything="mux 6-1 data") -> (Variant=w730:variant)
            n335 = call "App enquece.vi"("command data"=w730, "command"="MEAS.mux6_1", "queue in"=w731) -> ("error out"=w729:errorcluster)  [unwired: 7 in, 1 out]
            n336 = Merge Errors(w727, w729) -> (w728:errorcluster)
          }
          event "Mux 10-1": Value Change {
            n337 = event-data() -> ()  [unwired: 1 in, 1 out]
            n338 = disable-structure shown="LOGGING==TRUE" {
              disable-tunnel: w765 -> [w775 _]
              frame condition #0 (active) {
                n339 = Empty String/Path?(string/path=w775) -> (empty?=w782:bool)
                n340 = Select(t="Quece timeout", s=w782, f=w775) -> (s? t:f=w780:string)
                n341 = Format Into String(format string=": %s", initial string=w780, "mux10-1") -> (resulting string=w777:string)  [unwired: 1 in, 1 out]
                n342 = call "string log (SubVI).vi"("Enum"=enum16{"Init", "Log", "Read"}."Log", "state Name"=w777) -> ()  [unwired: 8 in, 2 out]
              }
              frame condition #1 {
              }
            }
            n343 = To Variant(anything="mux 10-1 data") -> (Variant=w770:variant)
            n344 = call "App enquece.vi"("command data"=w770, "command"="MEAS.mux10-1", "queue in"=w773) -> ("error out"=w767:errorcluster)  [unwired: 7 in, 1 out]
            n345 = Merge Errors(w768, w767) -> (w766:errorcluster)
          }
          event "request AC-all": Value Change {
            w789 = T8 {"eMIC 1"={"ACV"=0.0, "ACI"=0.0, "pF"=0.0, "kW"=0.0, "Freq"=0.0, "kvar"=0.0}, "eMIC 2"={"ACV"=0.0, "ACI"=0.0, "pF"=0.0, "kW"=0.0, "Freq"=0.0, "kvar"=0.0}, "eMIC 3"={"ACV"=0.0, "ACI"=0.0, "pF"=0.0, "kW"=0.0, "Freq"=0.0, "kvar"=0.0}, "eMIC 4"={"ACV"=0.0, "ACI"=0.0, "pF"=0.0, "kW"=0.0, "Freq"=0.0, "kvar"=0.0}, "eMIC 5"={"ACV"=0.0, "ACI"=0.0, "pF"=0.0, "kW"=0.0, "Freq"=0.0, "kvar"=0.0}, "eMIC 6"={"ACV"=0.0, "ACI"=0.0, "pF"=0.0, "kW"=0.0, "Freq"=0.0, "kvar"=0.0}}  # eMICs cluster
            n346 = event-data() -> ()  [unwired: 1 in, 1 out]
            n347 = disable-structure shown="LOGGING==TRUE" {
              disable-tunnel: w790 -> [w796 _]
              frame condition #0 (active) {
                n348 = Empty String/Path?(string/path=w796) -> (empty?=w803:bool)
                n349 = Select(t="Quece timeout", s=w803, f=w796) -> (s? t:f=w801:string)
                n350 = Format Into String(format string=": %s", initial string=w801, "request AC") -> (resulting string=w798:string)  [unwired: 1 in, 1 out]
                n351 = call "string log (SubVI).vi"("Enum"=enum16{"Init", "Log", "Read"}."Log", "state Name"=w798) -> ()  [unwired: 8 in, 2 out]
              }
              frame condition #1 {
              }
            }
            n352 = call "FGV wait for 6 eMICs.vi"("Enum"=enum16{"Init", "count"}."Init") -> ("error out"=w786:errorcluster)  [unwired: 8 in, 2 out]
            n353 = call "App enquece.vi"("error in (no error)"=w786, "command"="MEAS.requestAC", "queue in"=w795) -> ("error out"=w791:errorcluster)  [unwired: 7 in, 1 out]
            n354 = Merge Errors(w792, w791) -> (w788:errorcluster)
          }
          event User Event {
            n355 = event-data() -> ("Module ID"=w814:i32, "Array"=w829:T24[])  [unwired: 1 in]
            n356 = Variant To Data(type=0, Variant=w810) -> (data=w808:i32)  [unwired: 1 in, 1 out]
            n357 = for {
              tunnel: w829 -> [w892] mode=indexing
              shift-right: [w888] -> w805
              shift-left: T7 {"ACV"=0.0, "ACI"=0.0, "pF"=0.0, "kW"=0.0, "Freq"=0.0, "kvar"=0.0} ("eMIC response") -> [w890]
              n358 = Unbundle By Name(w892) -> ("float"=w889:dbl, "Name"=w891:string)
              n359 = case shown="\"kW\"" w891 {
                tunnel: w890 -> [w893 w896 w899 w902 w905 w908 w911]
                tunnel: w889 -> [_ w894 w897 w900 w904 w906 w910]
                tunnel: [w893 w895 w898 w901 w903 w907 w909] -> w888
                frame "False", Default {
                }
                frame "ACI" {
                  n360 = Bundle By Name(cluster=w896, "ACI"=w894) -> (w895:T7)
                }
                frame "kW" {
                  n361 = Bundle By Name(cluster=w899, "kW"=w897) -> (w898:T7)
                }
                frame "PF" {
                  n362 = Bundle By Name(cluster=w902, "pF"=w900) -> (w901:T7)
                }
                frame "ACV" {
                  n363 = Bundle By Name(cluster=w905, "ACV"=w904) -> (w903:T7)
                }
                frame "Freq" {
                  n364 = Bundle By Name(cluster=w908, "Freq"=w906) -> (w907:T7)
                }
                frame "kvar" {
                  n365 = Bundle By Name(cluster=w911, "kvar"=w910) -> (w909:T7)
                }
              }
            }
            n366 = disable-structure shown="LOGGING==TRUE" {
              disable-tunnel: w815 -> [w866 _]
              disable-tunnel: w814 -> [w862 _]
              frame condition #0 (active) {
                n367 = Empty String/Path?(string/path=w866) -> (empty?=w868:bool)
                n368 = Select(t="Quece timeout", s=w868, f=w866) -> (s? t:f=w865:string)
                n369 = Format Into String(format string=":%s %d", initial string=w865, "CE14  data response", w862) -> (resulting string=w861:string)  [unwired: 1 in, 1 out]
                n370 = call "string log (SubVI).vi"("Enum"=enum16{"Init", "Log", "Read"}."Log", "state Name"=w861) -> ()  [unwired: 8 in, 2 out]
              }
              frame condition #1 {
              }
            }
            n371 = call "eMIC_calibration.vi"("eMIC data in"=w805) -> ("eMIC data out"=w804:T7)  [unwired: 10 in]
            n372 = case shown="1" w814 {
              tunnel: [w869 w871 w874 w877 w880 w883 w886] -> w820
              tunnel: w821 -> [w869 w872 w875 w878 w881 w884 w887]
              tunnel: w804 -> [_ w870 w873 w876 w879 w882 w885]
              frame 0, Default {
              }
              frame 1 {
                n373 = Bundle By Name(cluster=w872, "eMIC 1"=w870) -> (w871:T8)
              }
              frame 2 {
                n374 = Bundle By Name(cluster=w875, "eMIC 2"=w873) -> (w874:T8)
              }
              frame 3 {
                n375 = Bundle By Name(cluster=w878, "eMIC 3"=w876) -> (w877:T8)
              }
              frame 4 {
                n376 = Bundle By Name(cluster=w881, "eMIC 4"=w879) -> (w880:T8)
              }
              frame 5 {
                n377 = Bundle By Name(cluster=w884, "eMIC 5"=w882) -> (w883:T8)
              }
              frame 6 {
                n378 = Bundle By Name(cluster=w887, "eMIC 6"=w885) -> (w886:T8)
              }
            }
            n379 = case shown="1, Default" w808 {
              tunnel: w820 -> [w837 w855]
              tunnel: w819 -> [w836 _]
              tunnel: [w834 w853] -> w816
              tunnel: w812 -> [w833 w859]
              tunnel: [w832 w859] -> w811
              tunnel: w807 -> [w831 w856]
              tunnel: [w831 w856] -> w806
              frame 0 {
                n380 = call "FGV wait for 6 eMICs.vi"("Enum"=enum16{"Init", "count"}."count") -> ("error out"=w835:errorcluster, "wait done"=w838:bool)  [unwired: 8 in, 1 out]
                "AC  Completed" <- w838
                n381 = case shown="True" w838 {
                  tunnel: w837 -> [_ w848]
                  tunnel: w833 -> [w840 w846]
                  tunnel: w836 -> [w845 _]
                  tunnel: w835 -> [w842 w850]
                  tunnel: [w841 w849] -> w834
                  tunnel: [w840 w846] -> w832
                  frame False {
                    n382 = call "App enquece.vi"("Priority Enquece"=TRUE, "error in (no error)"=w842, "command"="Apps.WaitForEvent", "queue in"=w845) -> ("error out"=w841:errorcluster)  [unwired: 6 in, 1 out]
                  }
                  frame True {
                    n383 = To Variant(anything=w848) -> (Variant=w847:variant)
                    n384 = call "FGV Driver Data.vi"("DUT channel (1-11)"=w846, "Mode"=DUT_data_Mode."AC parameter", "error in (no error)"=w850, "FGV enum(Read)"=FGV_DRV_data."Write" ("FGV DRV data enum"), "data"=w847) -> ("error out"=w849:errorcluster)  [unwired: 3 in, 3 out]
                  }
                }
              }
              frame 1, Default {
                n385 = To Variant(anything=w855) -> (Variant=w854:variant)
                n386 = call "FGV Driver Data.vi"("Mode"=DUT_data_Mode."AC parameter 1", "DUT index(1-60)"=w856, "FGV enum(Read)"=FGV_DRV_data."Write", "data"=w854) -> ("error out"=w853:errorcluster)  [unwired: 4 in, 3 out]
              }
            }
            n387 = Unbundle By Name(w820) -> ("eMIC 1"=→"eMIC 1":T7, "eMIC 2"=→"eMIC 2":T7, "eMIC 3"=→"eMIC 3":T7, "eMIC 4"=→"eMIC 4":T7, "eMIC 5"=→"eMIC 5":T7, "eMIC 6"=→"eMIC 6":T7)
            n388 = Merge Errors(w817, w816) -> (w818:errorcluster)
          }
          event User Event {
            n389 = event-data() -> ("Init?"=w925:bool, "Module ID"=w912:i32)  [unwired: 1 in]
            "Module ID" <- w912
            "AC Measure Module" <- w925
            n390 = disable-structure shown="LOGGING==TRUE" {
              disable-tunnel: w927 -> [w947 _]
              disable-tunnel: w912 -> [w943 _]
              frame condition #0 (active) {
                n391 = Empty String/Path?(string/path=w947) -> (empty?=w949:bool)
                n392 = Select(t="Quece timeout", s=w949, f=w947) -> (s? t:f=w946:string)
                n393 = Format Into String(format string=":%s %d", initial string=w946, "CE14 Did  it", w943) -> (resulting string=w942:string)  [unwired: 1 in, 1 out]
                n394 = call "string log (SubVI).vi"("Enum"=enum16{"Init", "Log", "Read"}."Log", "state Name"=w942) -> ()  [unwired: 8 in, 2 out]
              }
              frame condition #1 {
              }
            }
            n395 = disable-structure shown="DEBUGGING==TRUE" {
              disable-tunnel: w912 -> [w950 _]
              frame condition #0 {
                n396 = call "Show Panel.vi"("Module ID"=w950) -> ()  [unwired: 10 in, 1 out]
              }
              frame condition #1 (active) {
              }
            }
            n397 = Decrement(x=w912) -> (x-1=w926:i32)
            n398 = Initialize Array(FALSE, 6 ("dimension size")) -> (w921:bool[])
            n399 = feedback #2(w921) -> (w922:bool[])
            n400 = Replace Array Subset(array=w922, new element=w925, index=w926) -> (w920:bool[])
            "CE14  Module did it" <- w920
            n401 = feedback-in #2(w920) -> ()
            n402 = And Array Elements(Boolean array=w920) -> (logical AND=w919:bool)
            n403 = case shown="False" w919 {
              tunnel: w918 -> [_ w934]
              tunnel: [_ w933] -> w917
              frame False {
              }
              frame True {
                n404 = flat-sequence {
                  tunnel: [w936] -> w935
                  tunnel: w934 -> [w936]
                  tunnel: w935 -> [w939]
                  tunnel: [w938] -> w933
                  frame #0 {
                    n405 = Wait (ms)(milliseconds to wait=u32 500) -> ()  [unwired: 1 out]
                  }
                  frame #1 {
                    n406 = call "App enquece.vi"("command"="MEAS.Read EMIC connected", "queue in"=w939) -> ("error out"=w938:errorcluster)  [unwired: 8 in, 1 out]
                  }
                }
              }
            }
            n407 = control-ref of="Select CE14 eMIC Module Instance"() -> (w932:refnum<vi>)
            n408 = call "Update Select Module Ring.vi"("Select Module Ring Ref"=w932) -> ("error out"=w916:errorcluster)  [unwired: 8 in, 2 out]
            n409 = Merge Errors(w928, w917, w916) -> (w929:errorcluster)
          }
          event "Shorted Circuits Test": Value Change {
            n410 = event-data() -> ()  [unwired: 1 in, 1 out]
            n411 = Build Array("Test Shorted Circuits") -> (w956:string[])
            n412 = for {
              tunnel: [w968] -> w957 mode=indexing
              tunnel: w956 -> [w967] mode=indexing
              tunnel: w955 -> [w966]
              n413 = call "App enquece.vi"("command"=w967, "queue in"=w966) -> ("error out"=w968:errorcluster)  [unwired: 8 in, 1 out]
            }
            n414 = Merge Errors(w959, w957) -> (w958:errorcluster)
            n415 = disable-structure shown="Enabled" {
              frame Enabled {
                n416 = Initialize Array(FALSE, 6 ("dimension size"), 10 ("dimension size")) -> (w962:bool[][])
                n417 = local write "Short DRV"(w962) -> ()
              }
              frame Disabled {
              }
            }
          }
          event "Test Channel 1": Value Change {
            n418 = event-data() -> ()  [unwired: 1 in, 1 out]
            n419 = Array Subset(array=w976, index=0, length=6) -> (w973:refnum<vi>[])
            n420 = for {
              tunnel: w973 -> [w985] mode=indexing
              n421 = property class="ColBox"(reference=w985, "Value"=u32 10000536 ("DRV 1")) -> ()  [unwired: 1 in, 2 out]
            }
            n422 = Build Array("Test Channel 1", "MEAS.AllRelaysOFF") -> (w980:string[])
            n423 = for {
              tunnel: [w989] -> w981 mode=indexing
              tunnel: w980 -> [w988] mode=indexing
              tunnel: w979 -> [w987]
              n424 = call "App enquece.vi"("command"=w988, "queue in"=w987) -> ("error out"=w989:errorcluster)  [unwired: 8 in, 1 out]
            }
            n425 = Merge Errors(w983, w981) -> (w982:errorcluster)
          }
          event "Test Channel 2": Value Change {
            n426 = event-data() -> ()  [unwired: 1 in, 1 out]
            n427 = Array Subset(array=w995, index=6, length=6) -> (w994:refnum<vi>[])
            n428 = for {
              tunnel: w994 -> [w1006] mode=indexing
